vi "subSpeakerNote.vi"(6 "Volume":u8, 8 "error in":errorcluster, 9 "Note Duration (ms)":i32=400, 10 "Desired Freq":dbl, 11 "reference":refnum<k24>) -> (0 "error out":errorcluster, 3 "reference out":refnum<k24>)   [LabVIEW 2009]
uses:
  C:/Documents and Settings/ukbarnem/Desktop/project/Speaker Example/Resources/WiimoteLib.dll
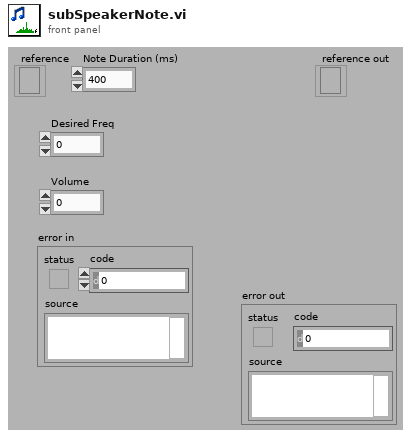
[diagram p1: front panel]
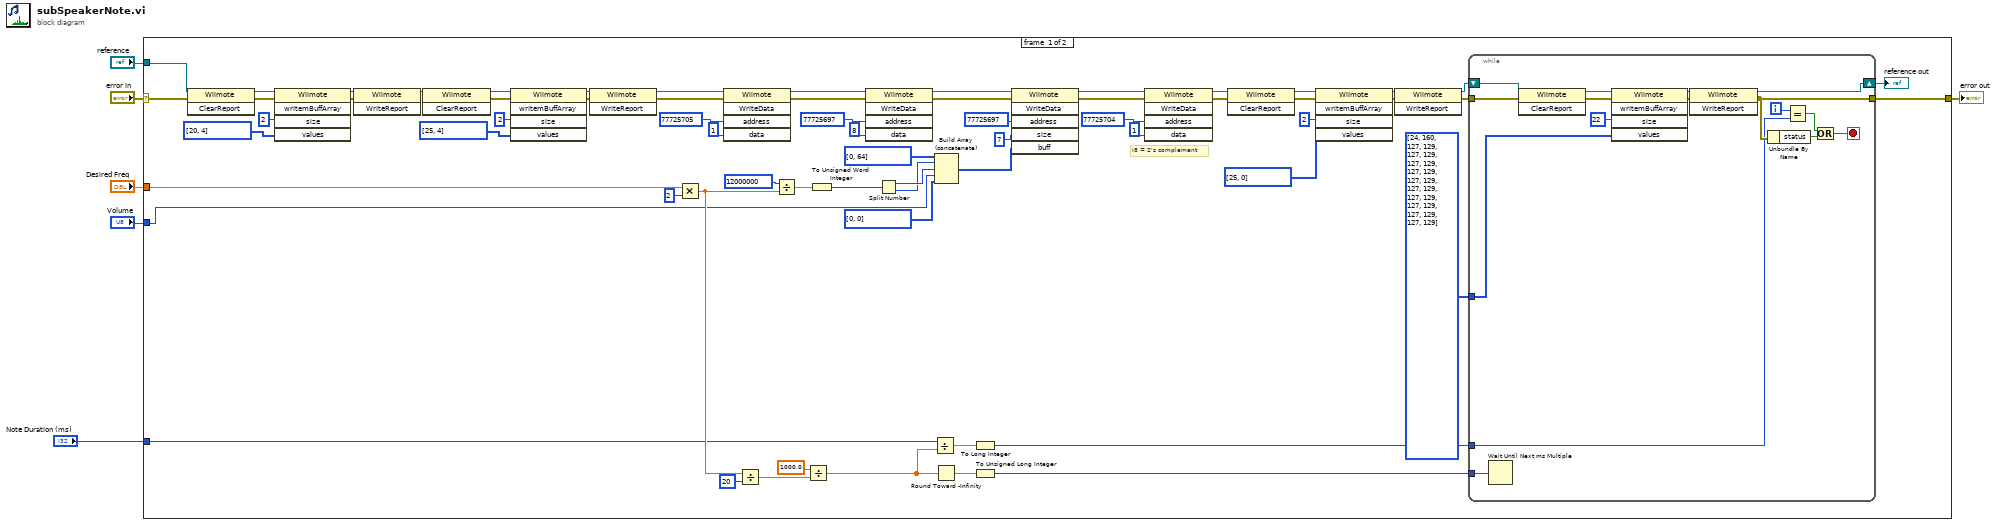
[diagram p0: block diagram]
diagram:
  n1 = case shown="No Error" "error in" {
    selector: "error in" -> [w12 w88]
    tunnel: [w15 w88] -> w6
    tunnel: "reference" -> [w11 _]
    tunnel: "Desired Freq" -> [w10 _]
    tunnel: "Note Duration (ms)" -> [w9 _]
    tunnel: "Volume" -> [w8 _]
    frame #0 {
      # "I8 = 2's complement"
      n2 = invoke class="Wiimote" method="ClearReport"(reference=w11, error in=w12) -> (reference out=w33:refnum<k24>, error out=w35:errorcluster)  [unwired: 1 in, 1 out]
      n3 = invoke class="Wiimote" method="writemBuffArray"(reference=w33, error in=w35, "size"=u8 2, "values"=u8[] [20, 4] ("Report Data")) -> (reference out=w34:refnum<k24>, error out=w36:errorcluster)  [unwired: 1 in, 3 out]
      n4 = invoke class="Wiimote" method="WriteReport"(reference=w34, error in=w36) -> (reference out=w31:refnum<k24>)  [unwired: 1 in, 2 out]
      n5 = invoke class="Wiimote" method="ClearReport"(reference=w31) -> (reference out=w43:refnum<k24>, error out=w41:errorcluster)  [unwired: 2 in, 1 out]
      n6 = invoke class="Wiimote" method="writemBuffArray"(reference=w43, error in=w41, "size"=u8 2, "values"=u8[] [25, 4] ("Report Data")) -> (reference out=w42:refnum<k24>, error out=w40:errorcluster)  [unwired: 1 in, 3 out]
      n7 = invoke class="Wiimote" method="WriteReport"(reference=w42, error in=w40) -> (reference out=w30:refnum<k24>, error out=w29:errorcluster)  [unwired: 1 in, 1 out]
      n8 = Multiply(x=w10, y=2) -> (x*y=w67:dbl)
      n9 = invoke class="Wiimote" method="WriteData"(reference=w30, error in=w29, "address"=77725705, "data"=u8 1) -> (reference out=w49:refnum<k24>, error out=w48:errorcluster)  [unwired: 1 in, 3 out]
      n10 = Divide(x=w67, y=20) -> (x/y=w69:dbl)
      n11 = Divide(x=12000000, y=w67) -> (x/y=w60:dbl)
      n12 = Divide(x=1000.0, y=w69) -> (x/y=w17:dbl)
      n13 = To Unsigned Word Integer(number=w60) -> (unsigned 16bit integer=w62:u16)
      n14 = invoke class="Wiimote" method="WriteData"(reference=w49, error in=w48, "address"=77725697, "data"=u8 8) -> (reference out=w50:refnum<k24>, error out=w51:errorcluster)  [unwired: 1 in, 3 out]
      n15 = Split Number(x=w62) -> (hi(x)=w64:u8, lo(x)=w63:u8)
      n16 = Divide(x=w9, y=w17) -> (x/y=w19:dbl)
      n17 = Round Toward -Infinity(1:w17) -> (0:w71:dbl)
      n18 = Build Array (concatenate)(u8[] [0, 64] ("buff"), w63, w64, w8, u8[] [0, 0] ("buff")) -> (w66:u8[])
      n19 = To Long Integer(number=w19) -> (32bit integer=w18:i32)
      n20 = To Unsigned Long Integer(number=w71) -> (unsigned 32bit integer=w20:u32)
      n21 = invoke class="Wiimote" method="WriteData"(reference=w50, error in=w51, "address"=77725697, "size"=u8 7, "buff"=w66) -> (reference out=w54:refnum<k24>, error out=w55:errorcluster)  [unwired: 1 in, 4 out]
      n22 = invoke class="Wiimote" method="WriteData"(reference=w54, error in=w55, "address"=77725704, "data"=u8 1) -> (reference out=w22:refnum<k24>, error out=w21:errorcluster)  [unwired: 1 in, 3 out]
      n23 = invoke class="Wiimote" method="ClearReport"(reference=w22, error in=w21) -> (reference out=w28:refnum<k24>, error out=w26:errorcluster)  [unwired: 1 in, 1 out]
      n24 = invoke class="Wiimote" method="writemBuffArray"(reference=w28, error in=w26, "size"=u8 2, "values"=u8[] [25, 0] ("Report Data")) -> (reference out=w27:refnum<k24>, error out=w25:errorcluster)  [unwired: 1 in, 3 out]
      n25 = invoke class="Wiimote" method="WriteReport"(reference=w27, error in=w25) -> (reference out=w14:refnum<k24>, error out=w16:errorcluster)  [unwired: 1 in, 1 out]
      n26 = while {
        tunnel: w16 -> [w82]
        tunnel: [w78] -> w15
        shift-right: [w81] -> w13
        shift-left: w14 -> [w83]
        tunnel: w18 -> [w75]
        tunnel: w20 -> [w74]
        tunnel: u8[] [24, 160, 127, 129, 127, 129, 127, 129, 127, 129, 127, 129, 127, 129, 127, 129, 127, 129, 127, 129, 127, 129] -> [w79]
        i -> [w76]
        stop <- w72 stop-if-true
        n27 = Wait Until Next ms Multiple(millisecond multiple=w74) -> ()  [unwired: 1 out]
        n28 = invoke class="Wiimote" method="ClearReport"(reference=w83, error in=w82) -> (reference out=w87:refnum<k24>, error out=w85:errorcluster)  [unwired: 1 in, 1 out]
        n29 = invoke class="Wiimote" method="writemBuffArray"(reference=w87, error in=w85, "size"=u8 22, "values"=w79) -> (reference out=w86:refnum<k24>, error out=w84:errorcluster)  [unwired: 1 in, 3 out]
        n30 = invoke class="Wiimote" method="WriteReport"(reference=w86, error in=w84) -> (reference out=w81:refnum<k24>, error out=w78:errorcluster)  [unwired: 1 in, 1 out]
        n31 = Unbundle By Name(w78) -> ("status"=w77:bool)
        n32 = Equal?(x=w76, y=w75) -> (x = y?=w73:bool)
        n33 = Or(x=w73, y=w77) -> (x .or. y?=w72:bool)
      }
      "reference out" <- w13
    }
    frame #1 {
    }
  }
  "error out" <- w6
